vi "曲线处理C.vi"(7 "基值":sgl=2.55 format="%.2f", 8 "历史数据":sgl[](array[numeric]), 11 "Pr":T1={"选择"=enum."Fx", "系数x"=1.0, "系数+"=1.0, "上限"=4.3, "下限"=3.7, "Ymax"=50.0, "Ymin"=-50.0, "点数"=1000.0, "锁系数x"=1.0, "锁上限"=0.4, "锁下限"=0.6, "锁系数+"=1.0, "起点"=0.20000000298023224, "终点"=0.6499999761581421, "锁起点"=0.05000000074505806, "锁终点"=0.20000000298023224, "上参考"=4.3, "下参考"=3.7, "基准"=3.7} {"系数+" format="%.3f"; "基准" format="%.2f"; "下参考" format="%.2f"; "上参考" format="%.2f"; "锁终点" format="%.2f"; "锁起点" format="%.2f"; "终点" format="%.2f"; "起点" format="%.2f"; "锁系数+" format="%.3f"; "锁下限" format="%.2f"; "锁上限" format="%.2f"; "锁系数x" format="%.3f"; "下限" format="%.2f"; "上限" format="%.2f"; "系数x" format="%.3f"}) -> (0 "范围内?":bool, 3 "曲线数组":sgl[](array[numeric]), 4 "示值+":string, 6 "示值":string)   [LabVIEW 2018]
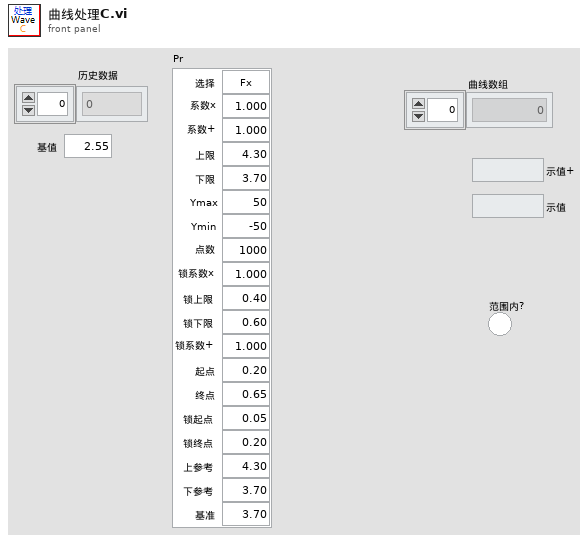
[diagram p1: front panel]
types:
  T1 = cluster{"选择":enum16{"Fx", "Fy", "Fz", "Mx", "My", "Mz"}, "系数x":sgl, "系数+":sgl, "上限":sgl, "下限":sgl, "Ymax":dbl, "Ymin":dbl, "点数":dbl, "锁系数x":sgl, "锁上限":sgl, "锁下限":sgl, "锁系数+":sgl, "起点":dbl, "终点":dbl, "锁起点":dbl, "锁终点":dbl, "上参考":sgl, "下参考":sgl, "基准":sgl}
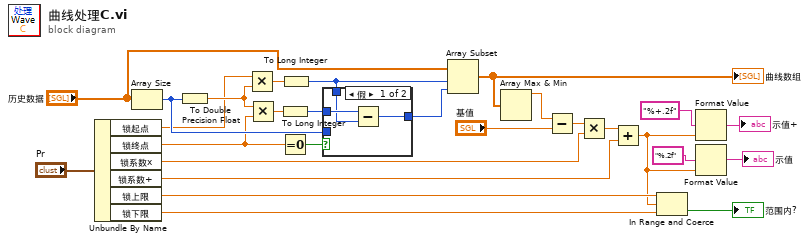
[diagram p0: block diagram]
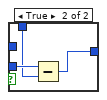
[diagram p2: hidden frame]
diagram:
  n1 = Unbundle By Name("Pr") -> ("锁起点"=w7:dbl, "锁终点"=w8:dbl, "锁系数x"=w13:sgl, "锁系数+"=w11:sgl, "锁上限"=w10:sgl, "锁下限"=w9:sgl)
  n2 = Array Size(array="历史数据") -> (size(s)=w20:i32)
  n3 = To Double Precision Float(number=w20) -> (double precision float=w18:dbl)
  n4 = Multiply(x=w7, y=w18) -> (x*y=w22:dbl)
  n5 = Multiply(x=w18, y=w8) -> (x*y=w21:dbl)
  n6 = To Long Integer(number=w21) -> (32bit integer=w19:i32)
  n7 = Equal To 0?(x=w8) -> (x = 0?=w23:bool)
  n8 = To Long Integer(number=w22) -> (32bit integer=w16:i32)
  n9 = case shown="假" w23 {
    tunnel: w20 -> [_ w33]
    tunnel: w19 -> [w30 _]
    tunnel: w16 -> [w29 w32]
    tunnel: [w28 w31] -> w15
    frame False {
      n10 = Subtract(x=w30, y=w29) -> (x-y=w28:i32)
    }
    frame True {
      n11 = Subtract(x=w33, y=w32) -> (x-y=w31:i32)
    }
  }
  n12 = Array Subset(array="历史数据", index=w16, length=w15) -> (w26:sgl[])
  "曲线数组" <- w26
  n13 = Array Max & Min(array=w26) -> (max value=w25:sgl)  [unwired: 3 out]
  n14 = Subtract(x=w25, y="基值") -> (x-y=w14:sgl)
  n15 = Multiply(x=w14, y=w13) -> (x*y=w12:sgl)
  n16 = Add(x=w12, y=w11) -> (x+y=w4:sgl)
  n17 = In Range and Coerce(upper limit=w10, x=w4, lower limit=w9) -> (In Range?=→"范围内?":bool)  [unwired: 1 out]
  n18 = Format Value(format string="%+.2f" ("格式字符串"), value (0)=w4) -> (output string=→"示值+":string)  [unwired: 1 in]
  n19 = Format Value(format string="%.2f" ("格式字符串"), value (0)=w4) -> (output string=→"示值":string)  [unwired: 1 in]
